vi "tree_move.vi"(10 "Left in":i32, 11 "Top":i32) -> (2 "Numeric":i32, 3 "Left out":dbl)   [LabVIEW 2022 SP3]
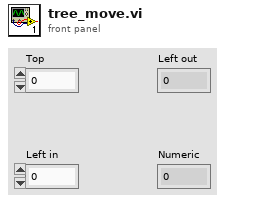
[diagram p1: front panel]
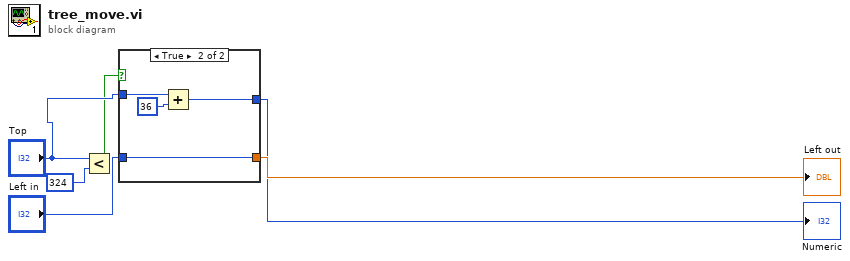
[diagram p0: block diagram]
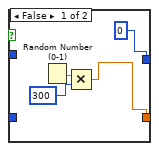
[diagram p2: hidden frame]
diagram:
  n1 = Less?(x="Top", y=324) -> (x < y?=w2:bool)
  n2 = case shown="True" w2 {
    tunnel: [0 w14] -> w5
    tunnel: "Top" -> [_ w13]
    tunnel: [w7 w11] -> w6
    tunnel: "Left in" -> [_ w11]
    frame False {
      n3 = Random Number (0-1)() -> (number: 0 to 1=w8:dbl)
      n4 = Multiply(x=w8, y=300) -> (x*y=w7:dbl)
    }
    frame True {
      n5 = Add(x=w13, y=36) -> (x+y=w14:i32)
    }
  }
  "Left out" <- w6
  "Numeric" <- w5
